vi "Save_double_Big_Array_to_Excel_copy.vi"(8 "에러 입력(에러 없음)":errorcluster, 9 "start (0, 0)":cluster{"row":i32, "column":i32}, 10 "배열":dbl[](array[numeric]) format="%#_9g", 11 "NI_report 입력":refnum<class "NI_report.lvclass">) -> (0 "error out":errorcluster, 1 "Next Position":cluster{"row":i32, "column":i32}, 3 "report out":refnum<class "NI_report.lvclass">)   [LabVIEW 2015]
uses:
  <vilib>/Utility/NIReport.llb/NI_report.lvclass
  <vilib>/addons/_office/excel.llb/Excel Easy Table (num).vi
  <vilib>/addons/_office/NI_ReportGenerationToolkit.lvlib
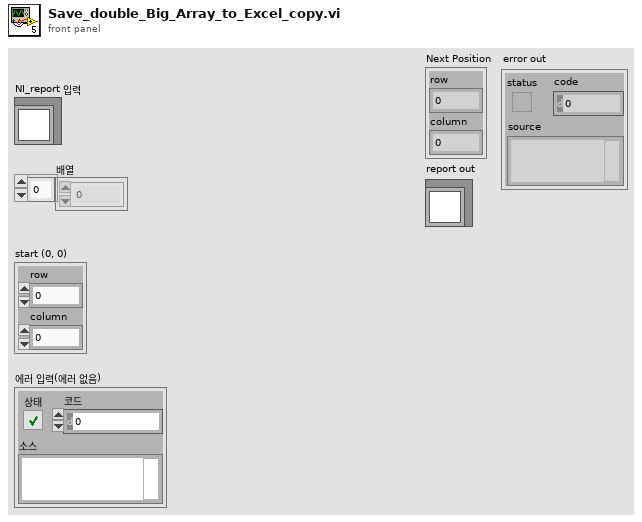
[diagram p1: front panel]
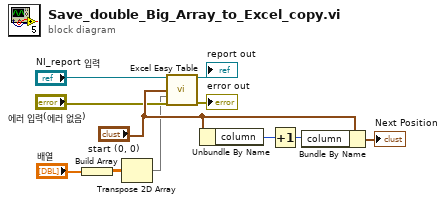
[diagram p0: block diagram]
diagram:
  n1 = Build Array("배열") -> (w2:dbl[][])
  n2 = Transpose 2D Array(2D array=w2) -> (transposed array=w1:dbl[][])
  n3 = call-poly <vilib>:"Excel Easy Table.vi"("report in"="NI_report 입력", "start (0, 0)"="start (0, 0)", "text data"=w1, "error in (no error)"="에러 입력(에러 없음)") -> ("report out"=→"report out":refnum<class "NI_report.lvclass">, "error out"=→"error out":errorcluster)  [unwired: 7 in, 3 out]
  n4 = Unbundle By Name("start (0, 0)") -> ("column"=w10:i32)
  n5 = Increment(x=w10) -> (x+1=w11:i32)
  n6 = Bundle By Name(cluster="start (0, 0)", "column"=w11) -> (→"Next Position":cluster{"row":i32, "column":i32})
